vi "ParFileString.vi"(1 "Trigger Levels":i16[](array[numeric]), 3 "number of readouts per file":u32=1000, 4 "Read Size":u32=750000 format="%.2p", 5 "# of pretrigger":u32=20, 6 "Record Size\nonly data":u32=95) -> (0 "Info in .par file":string)   [LabVIEW 2012]
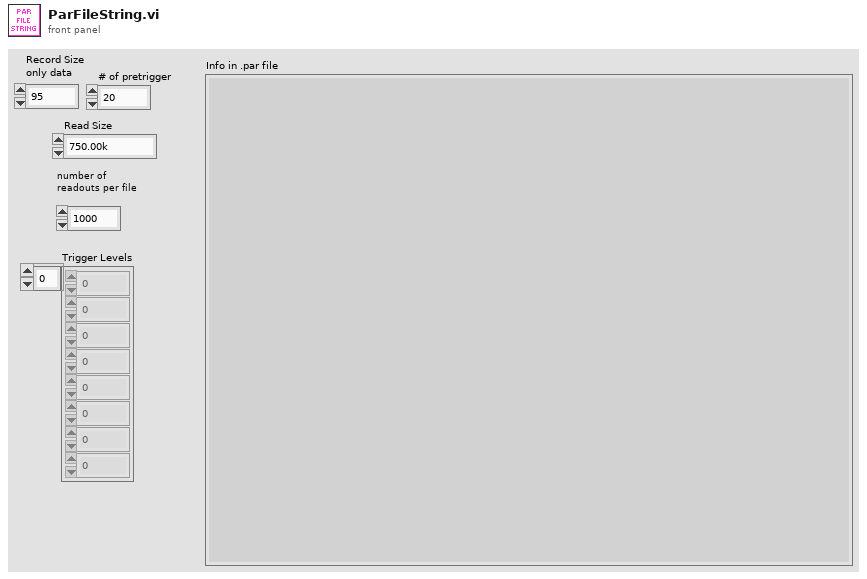
[diagram p1: front panel]
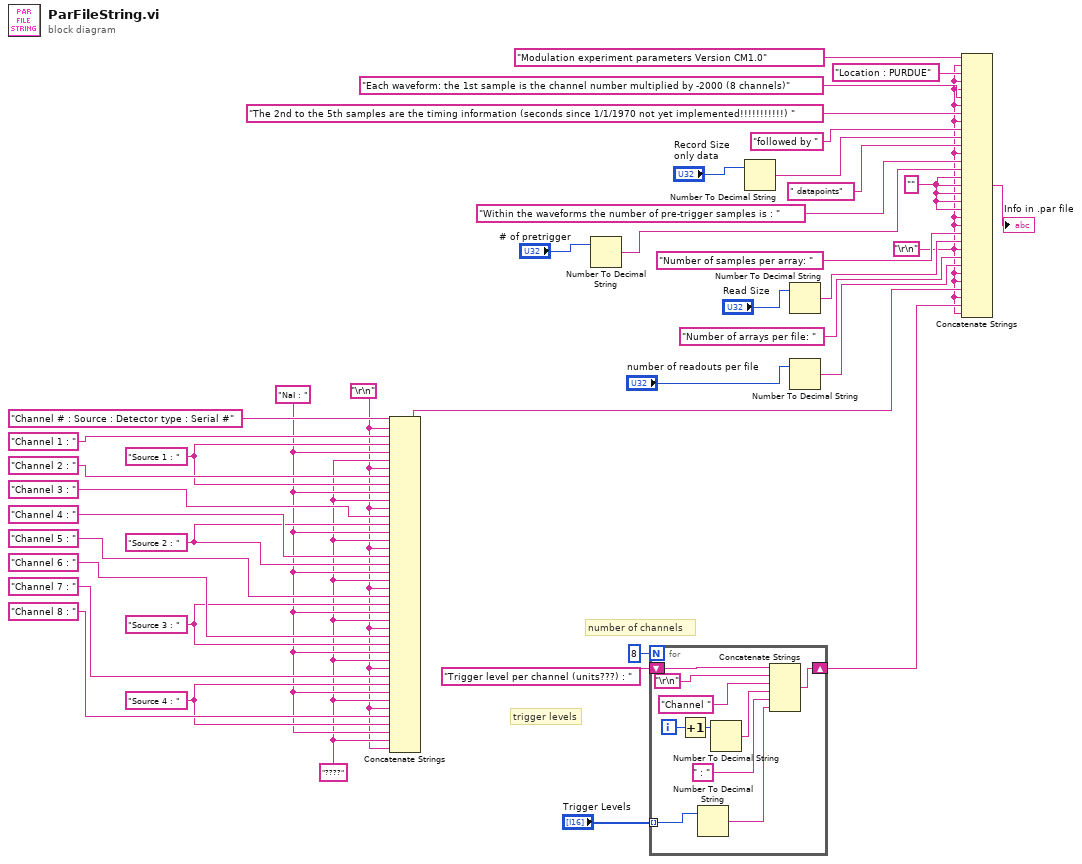
[diagram p0: block diagram]
diagram:
  w17 = "????" ("string")
  w18 = "NaI : " ("string")
  w16 = "\r\n"
  w19 = "Source 4 : " ("string")
  w22 = "Source 3 : " ("string")
  w25 = "Source 2 : " ("string")
  w28 = "Source 1 : " ("string")
  w6 = "" ("string")
  w1 = "\r\n"
  # "trigger levels"
  # "number of channels"
  n1 = Concatenate Strings("Channel # : Source : Detector type : Serial #" ("string"), w16, "Channel 1 : " ("string"), w28, w18, w17, w16, "Channel 2 : " ("string"), w28, w18, w17, w16, "Channel 3 : " ("string"), w25, w18, w17, w16, "Channel 4 : " ("string"), w25, w18, w17, w16, "Channel 5 : " ("string"), w22, w18, w17, w16, "Channel 6 : " ("string"), w22, w18, w17, w16, "Channel 7 : " ("string"), w19, w18, w17, w16, "Channel 8 : " ("string"), w19, w18, w17, w16) -> (w15:string)
  n2 = Number To Decimal String(number="# of pretrigger") -> (decimal integer string=w7:string)  [unwired: 1 in]
  n3 = for {
    N: 8 -> [_]
    tunnel: "Trigger Levels" -> [w51] mode=indexing
    shift-right: [w42] -> w2
    shift-left: "Trigger level per channel (units???) : " -> [w50]
    i -> [w47]
    n4 = Increment(x=w47) -> (x+1=w46:i32)
    n5 = Number To Decimal String(number=w51) -> (decimal integer string=w43:string)  [unwired: 1 in]
    n6 = Number To Decimal String(number=w46) -> (decimal integer string=w45:string)  [unwired: 1 in]
    n7 = Concatenate Strings(w50, "\r\n", "Channel " ("string"), w45, " : " ("string"), w43) -> (w42:string)
  }
  n8 = Number To Decimal String(number="Record Size\nonly data") -> (decimal integer string=w11:string)  [unwired: 1 in]
  n9 = Number To Decimal String(number="Read Size") -> (decimal integer string=w39:string)  [unwired: 1 in]
  n10 = Number To Decimal String(number="number of readouts per file") -> (decimal integer string=w38:string)  [unwired: 1 in]
  n11 = Concatenate Strings("Modulation experiment parameters Version CM1.0", w1, "Location : PURDUE" ("string"), w1, w1, "Each waveform: the 1st sample is the channel number multiplied by -2000 (8 channels)" ("string"), w1, "The 2nd to the 5th samples are the timing information (seconds since 1/1/1970 not yet implemented!!!!!!!!!!!) " ("string"), w1, "followed by " ("string"), w11, " datapoints" ("string"), w1, "Within the waveforms the number of pre-trigger samples is : " ("string"), w7, w6, w6, w6, w6, w6, w1, w1, "Number of samples per array: " ("string"), w39, w1, "Number of arrays per file: " ("string"), w38, w1, w1, w15, w1, w2, w1) -> (→"Info in .par file":string)
